vi "set_data_folder_path.vi"(8 "error in (no error)":errorcluster, 10 "data folder path":path, 11 "GenericComponent in":refnum<class "GenericComponent.lvclass">) -> (0 "error out":errorcluster, 3 "GenericComponent out":refnum<class "GenericComponent.lvclass">)   [LabVIEW 2010, in "GenericComponent.lvclass"]
uses:
  GenericComponent.lvclass
  class_data.vi
  NoteBook/Notebook/Notebook.lvclass
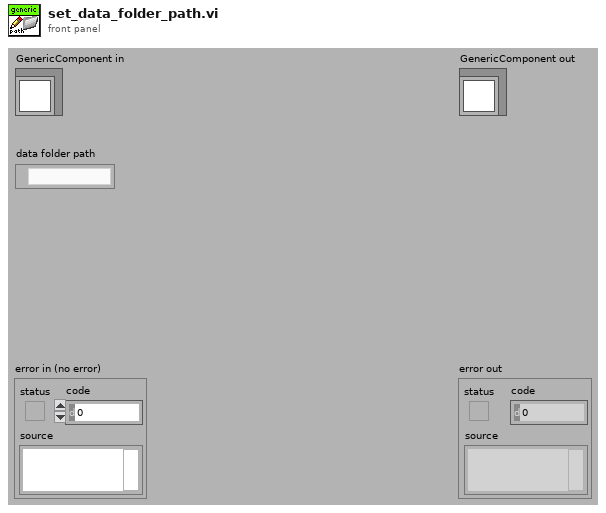
[diagram p1: front panel]
types:
  T1 = typedef "controls_refs.ctl" = cluster{"scan start button":refnum<vi>, "tabs":cluster{"main":refnum<vi>, "settings":refnum<vi>}, "subpanels":cluster{"imagingMode":refnum<vi>, "scanHead":refnum<vi>, "display":refnum<vi>, "experimentController":refnum<vi>, "instrument":refnum<vi>, "stage":refnum<vi>, "stimulator":refnum<vi>, "dataCollection":refnum<vi>, "analyser":refnum<vi>, "daq":refnum<vi>, "imageAssembler":refnum<vi>}, "drop-downs":cluster{"run mode":refnum<vi>, "imagingMode":refnum<vi>, "experimentalController":refnum<vi>, "objective":refnum<vi>}, "status lights":cluster{"experimentController":refnum<vi>, "imagingMode":refnum<vi>, "scanHead":refnum<vi>, "daq":refnum<vi>, "imageAssembler":refnum<vi>, "dataCollection":refnum<vi>, "display":refnum<vi>, "analyser":refnum<vi>, "stage":refnum<vi>, "stimulator":refnum<vi>, "instrument":refnum<vi>}, "message":refnum<vi>, "stimulator enabled?":refnum<vi>, "saving":cluster{"data folder path":refnum<vi>, "file base name":refnum<vi>, "notebook":refnum<vi>}, "progress bar":refnum<vi>, "update icon":refnum<vi>, "title":refnum<vi>, "main vi":refnum<vi>, "user":refnum<vi>, "exit_button":refnum<vi>, "CPU usage %":refnum<vi>}
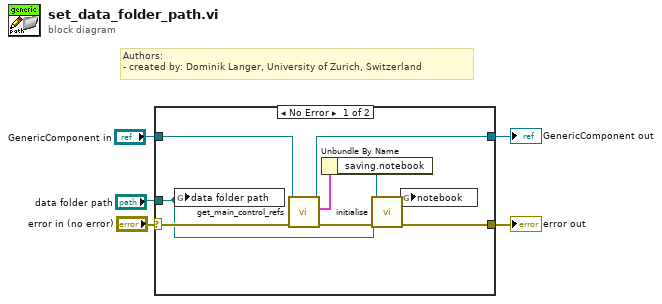
[diagram p0: block diagram]
diagram:
  # "Authors: \n- created by: Dominik Langer, University of Zurich, Switzerland"
  n1 = case shown="No Error" "error in (no error)" {
    selector: "error in (no error)" -> [w7 w16]
    tunnel: [w14 w16] -> w4
    tunnel: [w11 w15] -> w2
    tunnel: "GenericComponent in" -> [w12 w15]
    tunnel: "data folder path" -> [w6 _]
    frame No Error {
      n2 = global write "class_data.vi" "data folder path"(w6) -> ()
      n3 = call-dynamic "get_main_control_refs.vi"("error in (no error)"=w7, "GenericPlugin.lvclass in"=w12) -> ("error out"=w10:errorcluster, "control references"=w9:T1, "GenericPlugin.lvclass out"=w11:refnum<class "GenericComponent.lvclass">)  [unwired: 7 in]
      n4 = Unbundle By Name(w9) -> ("saving.notebook"=w8:refnum<vi>)
      n5 = call "initialise.vi"("error in (no error)"=w10, "folder path"=w6, "notebook control ref"=w8) -> ("error out"=w14:errorcluster, "Notebook out"=w13:refnum<class "Notebook.lvclass">)  [unwired: 7 out]
      n6 = global write "class_data.vi" "notebook"(w13) -> ()
    }
    frame Error {
    }
  }
  "error out" <- w4
  "GenericComponent out" <- w2
